vi "Print Popup.vi"(8 "error in":errorcluster, 11 "queue in":refnum<queue>) -> (0 "error out":errorcluster, 3 "queue out":refnum<queue>)   [LabVIEW 2024]
panel:
  out "Saved to:":string
  out "Progress (popup)":u8(slide) caption="Horizontal Slider" scale=0.0..100.0
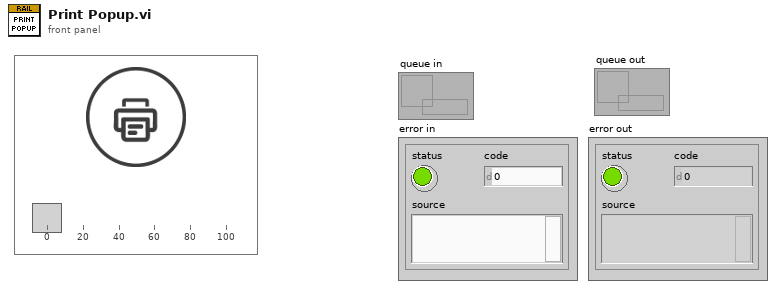
[diagram p1: front panel]
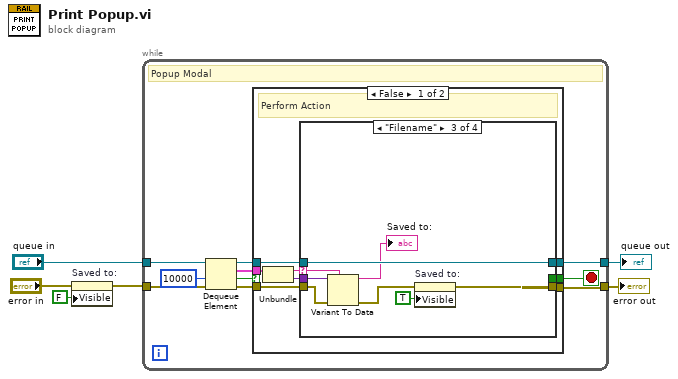
[diagram p0: block diagram]
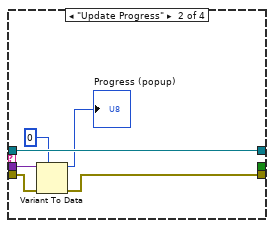
[diagram p3: hidden frame]
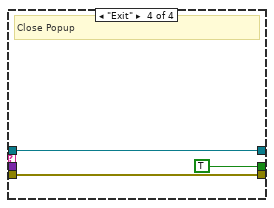
[diagram p4: hidden frame]
diagram:
  n1 = property on="Saved to:" class="Str"(error in="error in", "Visible"=FALSE) -> (error out=w2:errorcluster)  [unwired: 1 in, 1 out]
  n2 = while {
    tunnel: w2 -> [w15]
    tunnel: "queue in" -> [w16]
    tunnel: [w8] -> w6
    tunnel: [w7] -> w4
    stop <- w9 stop-if-true
    # "Popup Modal"
    n3 = Dequeue Element(queue=w16, timeout in ms (-1)=10000, error in (no error)=w15) -> (queue out=w11:refnum<queue>, element=w13:cluster{"Command":string, "Data":variant}, timed out?=w10:bool, error out=w12:errorcluster)
    n4 = case shown="False" w10 {
      selector: w10 -> [_ w46]
      tunnel: w13 -> [w24 _]
      tunnel: w12 -> [w23 w44]
      tunnel: w11 -> [w22 w45]
      tunnel: [w21 w46] -> w9
      tunnel: [w20 w44] -> w8
      tunnel: [w19 w45] -> w7
      frame False {
        # "Perform Action"
        n5 = Unbundle(w24) -> ("Command"=w18:string, "Data"=w17:variant)
        n6 = case shown="\"Filename\"" w18 {
          selector: w18 -> [_ _ w37 _]
          tunnel: w23 -> [w25 w30 w38 w42]
          tunnel: w22 -> [w26 w32 w40 w41]
          tunnel: [_ _ _ TRUE] -> w21
          tunnel: [w25 w29 w33 w42] -> w20
          tunnel: [w26 w32 w40 w41] -> w19
          tunnel: w17 -> [_ w31 w39 _]
          frame "False", Default {
          }
          frame "Update Progress" {
            n7 = Variant To Data(error in=w30, type=u8 0, Variant=w31) -> (data=→"Progress (popup)":u8, error out=w29:errorcluster)
          }
          frame "Filename" {
            n8 = Variant To Data(error in=w38, type=w37, Variant=w39) -> (data=→"Saved to:":string, error out=w34:errorcluster)
            n9 = property on="Saved to:" class="Str"(error in=w34, "Visible"=TRUE) -> (error out=w33:errorcluster)  [unwired: 1 in, 1 out]
          }
          frame "Exit" {
            # "Close Popup"
          }
        }
      }
      frame True {
        # "Timed out... some problem, so exit"
      }
    }
  }
  "error out" <- w6
  "queue out" <- w4
